vi "oax_Sync DSA and TIO (DAQmx).vi"(4 "Slave Slot Number":i32(ring) caption="PXI Slot Number" items=["Slot 3", "Slot 4", "Slot 5", "Slot 6", "Slot 7", "Slot 8", "Slot 9", "Slot 10", "Slot 11", "Slot 12", "Slot 13", "Slot 14", "Slot 15", "Slot 16"], 6 "DSA device type":u16(ring) items=["447x", "446x"], 8 "error in":errorcluster, 10 "TIO task in":refnum<k21>, 11 "DSA task in":refnum<k21>) -> (0 "error in":errorcluster, 2 "TIO task out":refnum<k21>, 3 "DSA task out":refnum<k21>)   [LabVIEW 2017]
uses:
  <resource>/objmgr/daqmx.rc
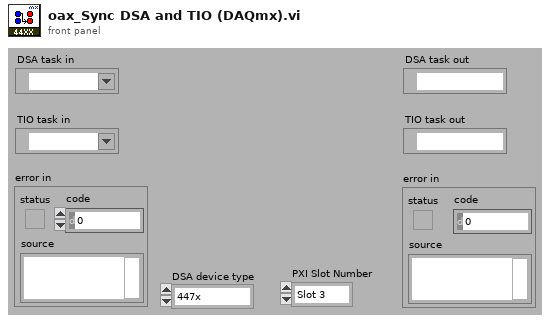
[diagram p1: front panel]
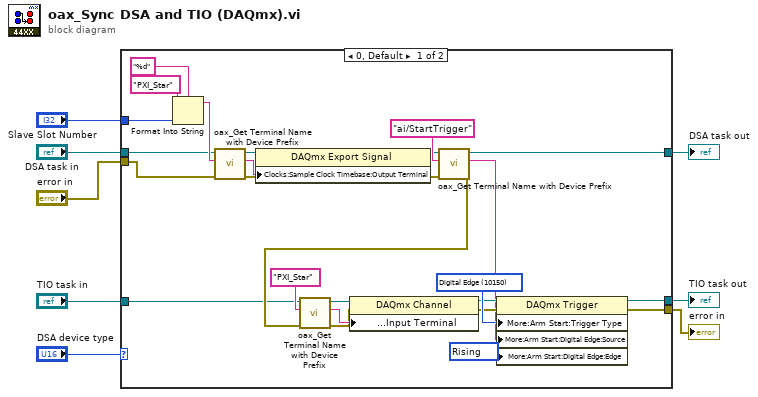
[diagram p0: block diagram]
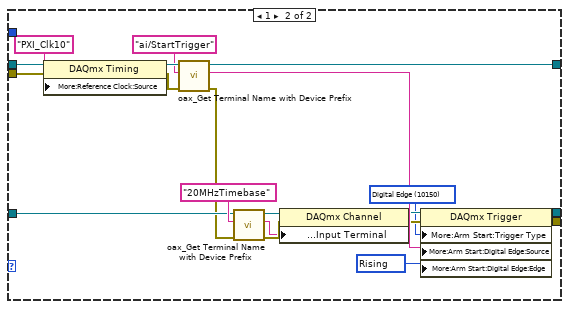
[diagram p2: hidden frame]
diagram:
  n1 = case shown="0, Default" "DSA device type" {
    tunnel: [w11 w54] -> w8
    tunnel: "DSA task in" -> [w17 w49]
    tunnel: "TIO task in" -> [w13 w42]
    tunnel: [w9 w39] -> w5
    tunnel: [w10 w38] -> w4
    tunnel: "error in" -> [w16 w36]
    tunnel: "Slave Slot Number" -> [w15 _]
    frame 0, Default {
      w24 = 10280 items=["Rising"=10280, "Falling"=10171] ("ArmStart.DigEdge.Edge")
      w25 = 10150 items=["Digital Edge"=10150, "None"=10230] ("ArmStart.TrigType")
      n2 = Format Into String(format string="%d", initial string="PXI_Star", w15) -> (resulting string=w26:string)  [unwired: 1 in, 1 out]
      n3 = call <vilib>:"oax_Get Terminal Name with Device Prefix.vi"("error in (no error)"=w16, "Local Terminal Name"=w26, "task/channels in"=w17) -> ("error out"=w30:errorcluster, "Terminal Name with Device Prefix"=w27:tag, "task out"=w31:refnum<k21>)  [unwired: 6 in]
      n4 = property class="DAQmx Export Signal"(reference=w31, error in=w30, "Clocks:Sample Clock Timebase:Output Terminal"=w27) -> (reference out=w29:refnum<k21>, error out=w28:errorcluster)
      n5 = call <vilib>:"oax_Get Terminal Name with Device Prefix.vi"("error in (no error)"=w28, "Local Terminal Name"="ai/StartTrigger", "task/channels in"=w29) -> ("error out"=w14:errorcluster, "Terminal Name with Device Prefix"=w12:tag, "task out"=w11:refnum<k21>)  [unwired: 6 in]
      n6 = call <vilib>:"oax_Get Terminal Name with Device Prefix.vi"("error in (no error)"=w14, "Local Terminal Name"="PXI_Star", "task/channels in"=w13) -> ("error out"=w20:errorcluster, "Terminal Name with Device Prefix"=w21:tag, "task out"=w22:refnum<k21>)  [unwired: 6 in]
      n7 = property class="DAQmx Channel"(reference=w22, error in=w20, "Counter Input:Count Edges:Input Terminal"=w21) -> (reference out=w19:refnum<k21>, error out=w18:errorcluster)
      n8 = property class="DAQmx Trigger"(reference=w19, error in=w18, "More:Arm Start:Trigger Type"=w25, "More:Arm Start:Digital Edge:Source"=w12, "More:Arm Start:Digital Edge:Edge"=w24) -> (reference out=w10:refnum<k21>, error out=w9:errorcluster)
    }
    frame 1 {
      w41 = 10280 items=["Rising"=10280, "Falling"=10171] ("ArmStart.DigEdge.Edge")
      w40 = 10150 items=["Digital Edge"=10150, "None"=10230] ("ArmStart.TrigType")
      n9 = property class="DAQmx Timing"(reference=w49, error in=w36, "More:Reference Clock:Source"="PXI_Clk10" ("Local Terminal Name")) -> (reference out=w50:refnum<k21>, error out=w51:errorcluster)
      n10 = call <vilib>:"oax_Get Terminal Name with Device Prefix.vi"("error in (no error)"=w51, "Local Terminal Name"="ai/StartTrigger", "task/channels in"=w50) -> ("error out"=w35:errorcluster, "Terminal Name with Device Prefix"=w48:tag, "task out"=w54:refnum<k21>)  [unwired: 6 in]
      n11 = call <vilib>:"oax_Get Terminal Name with Device Prefix.vi"("error in (no error)"=w35, "Local Terminal Name"="20MHzTimebase", "task/channels in"=w42) -> ("error out"=w45:errorcluster, "Terminal Name with Device Prefix"=w44:tag, "task out"=w43:refnum<k21>)  [unwired: 6 in]
      n12 = property class="DAQmx Channel"(reference=w43, error in=w45, "Counter Input:Count Edges:Input Terminal"=w44) -> (reference out=w46:refnum<k21>, error out=w47:errorcluster)
      n13 = property class="DAQmx Trigger"(reference=w46, error in=w47, "More:Arm Start:Trigger Type"=w40, "More:Arm Start:Digital Edge:Source"=w48, "More:Arm Start:Digital Edge:Edge"=w41) -> (reference out=w38:refnum<k21>, error out=w39:errorcluster)
    }
  }
  "DSA task out" <- w8
  "error in" <- w5
  "TIO task out" <- w4
